vi "loadDataToBuffer.vi"(8 "error in (no error)":errorcluster, 11 "K2602 in":refnum<class "K2602.lvclass">) -> (0 "error out":errorcluster, 3 "K2602 out":refnum<class "K2602.lvclass">)   [LabVIEW 2011, in "Hardware.lvlib" / "Channels.lvlib" / "K2602.lvclass"]
doc: "Abstract Method.\n\nThis vi, via its implementing classes, loads the analog output data to the buffer of the device."
uses:
  K2602.lvclass
  AnalogOutput.lvclass
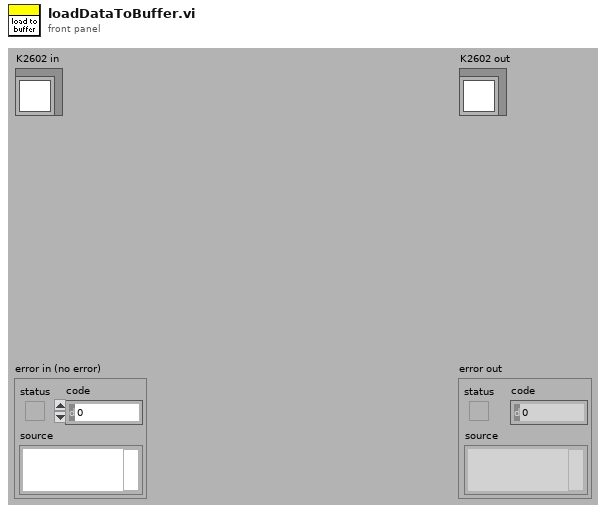
[diagram p1: front panel]
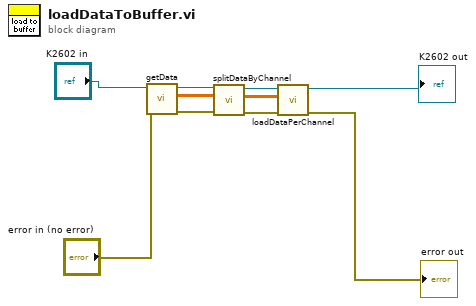
[diagram p0: block diagram]
diagram:
  n1 = call "getData.vi"("error in (no error)"="error in (no error)", "AnalogOutput.lvclass in"="K2602 in") -> ("error out"=w6:errorcluster, "Data"=w8:dbl[][], "AnalogOutput.lvclass out"=w9:refnum<class "K2602.lvclass">)  [unwired: 7 in]
  n2 = call "splitDataByChannel.vi"("error in (no error)"=w6, "Data"=w8, "K2602 in"=w9) -> ("error out"=w3:errorcluster, "data"=w4:dbl[][][], "K2602 out"=w5:refnum<class "K2602.lvclass">)  [unwired: 6 in]
  n3 = call-dynamic "loadDataPerChannel.vi"("error in (no error)"=w3, "data"=w4, "K2602 in"=w5) -> ("error out"=→"error out":errorcluster, "K2602 out"=→"K2602 out":refnum<class "K2602.lvclass">)  [unwired: 7 in]
